vi "Get Control Reference by Label (0D STR).vi"(8 "error in (no error)":errorcluster, 10 "Control Name":string, 11 "Control Ref Map":map{string, refnum<vi>}(c390)) -> (0 "error out":errorcluster, 2 "Found?":bool, 3 "Control Ref":refnum<vi>)   [LabVIEW 2020, in "MacroAssert.lvlib"]
doc: "Gets the reference of <B>Control Name</B> from <B>Control Ref Map</B>."
uses:
  MacroAssert.lvlib
  <vilib>/Utility/error.llb/Error Cluster From Error Code.vi
  SubVIs/Custom Errors/Custom Errors.lvlib
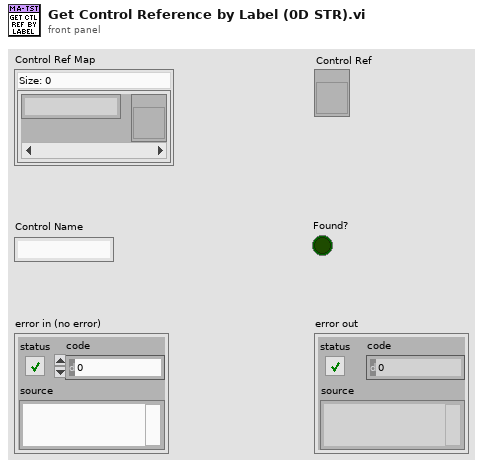
[diagram p1: front panel]
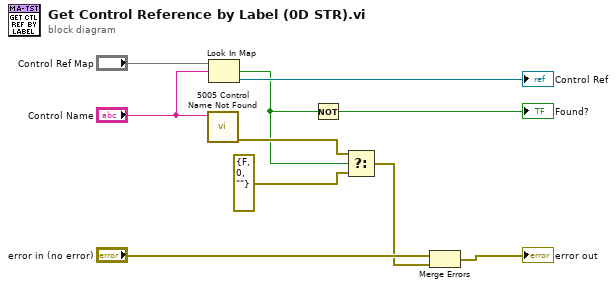
[diagram p0: block diagram]
diagram:
  n1 = call "5005 Control Name Not Found.vi"("Control Name"="Control Name") -> ("error out"=w5:errorcluster)  [unwired: 10 in]
  n2 = Look In Map(map="Control Ref Map", key="Control Name") -> (key not found?=w2:bool, value=→"Control Ref":refnum<vi>)  [unwired: 1 in]
  n3 = Not(x=w2) -> (.not. x?=→"Found?":bool)
  n4 = Select(t=w5, s=w2, f=errorcluster {"status"=FALSE, "code"=0, "source"=""} ("error in (no error)")) -> (s? t:f=w3:errorcluster)
  n5 = Merge Errors("error in (no error)", w3) -> (→"error out":errorcluster)
